vi "New JSON Array (Boolean).vi"(8 "error in (no error)":errorcluster, 10 "Boolean Array":bool[](array[boolean])) -> (0 "error out":errorcluster, 3 "JSON Value out":refnum<class "JSON Value.lvclass">)   [LabVIEW 2016, in "JSON Value.lvclass"]
doc: "Creates a new JSON Array initialized with JSON Boolean objects of the values specified by Boolean Array"
uses:
  JSON Value.lvclass
  New JSON Boolean.vi
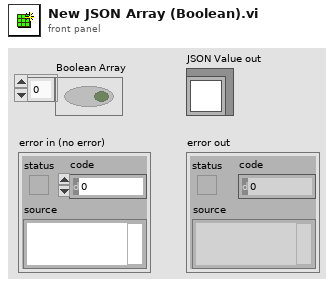
[diagram p1: front panel]
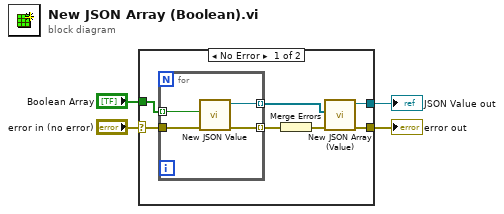
[diagram p0: block diagram]
diagram:
  n1 = case shown="No Error" "error in (no error)" {
    selector: "error in (no error)" -> [w7 w16]
    tunnel: [w9 w16] -> w3
    tunnel: [w8 _] -> w2
    tunnel: "Boolean Array" -> [w11 _]
    frame No Error {
      n2 = for {
        tunnel: w11 -> [w15] mode=indexing
        tunnel: [w14] -> w10 mode=indexing
        tunnel: w7 -> [w13]
        tunnel: [w12] -> w6 mode=indexing
        n3 = call-poly "New JSON Value.vi"("error in (no error)"=w13, "value"=w15) -> ("error out"=w12:errorcluster, "JSON Value out"=w14:refnum<class "JSON Value.lvclass">)  [unwired: 8 in]
      }
      n4 = Merge Errors(w6) -> (w5:errorcluster)
      n5 = call "New JSON Array (Value).vi"("error in (no error)"=w5, "JSON Datatypes"=w10) -> ("error out"=w9:errorcluster, "JSON Value out"=w8:refnum<class "JSON Value.lvclass">)  [unwired: 8 in]
    }
    frame Error {
    }
  }
  "error out" <- w3
  "JSON Value out" <- w2
